vi "HW 2-1.vi"() -> ()   [LabVIEW 2017]
panel:
  in  "%":bool
  in  "+/-":bool
  in  ".":bool
  in  "blackspace":bool
  in  "ce":bool
  in  "c":bool
  in  "/":bool
  out "String":string
  in  "=":bool
  in  "c":bool
  in  "*":bool
  in  "-":bool
  in  "+":bool
  in  "9":bool
  in  "8":bool
  in  "7":bool
  in  "6":bool
  in  "5":bool
  in  "4":bool
  in  "3":bool
  in  "2":bool
  in  "1":bool
  in  "0":bool
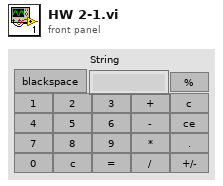
[diagram p1: front panel]
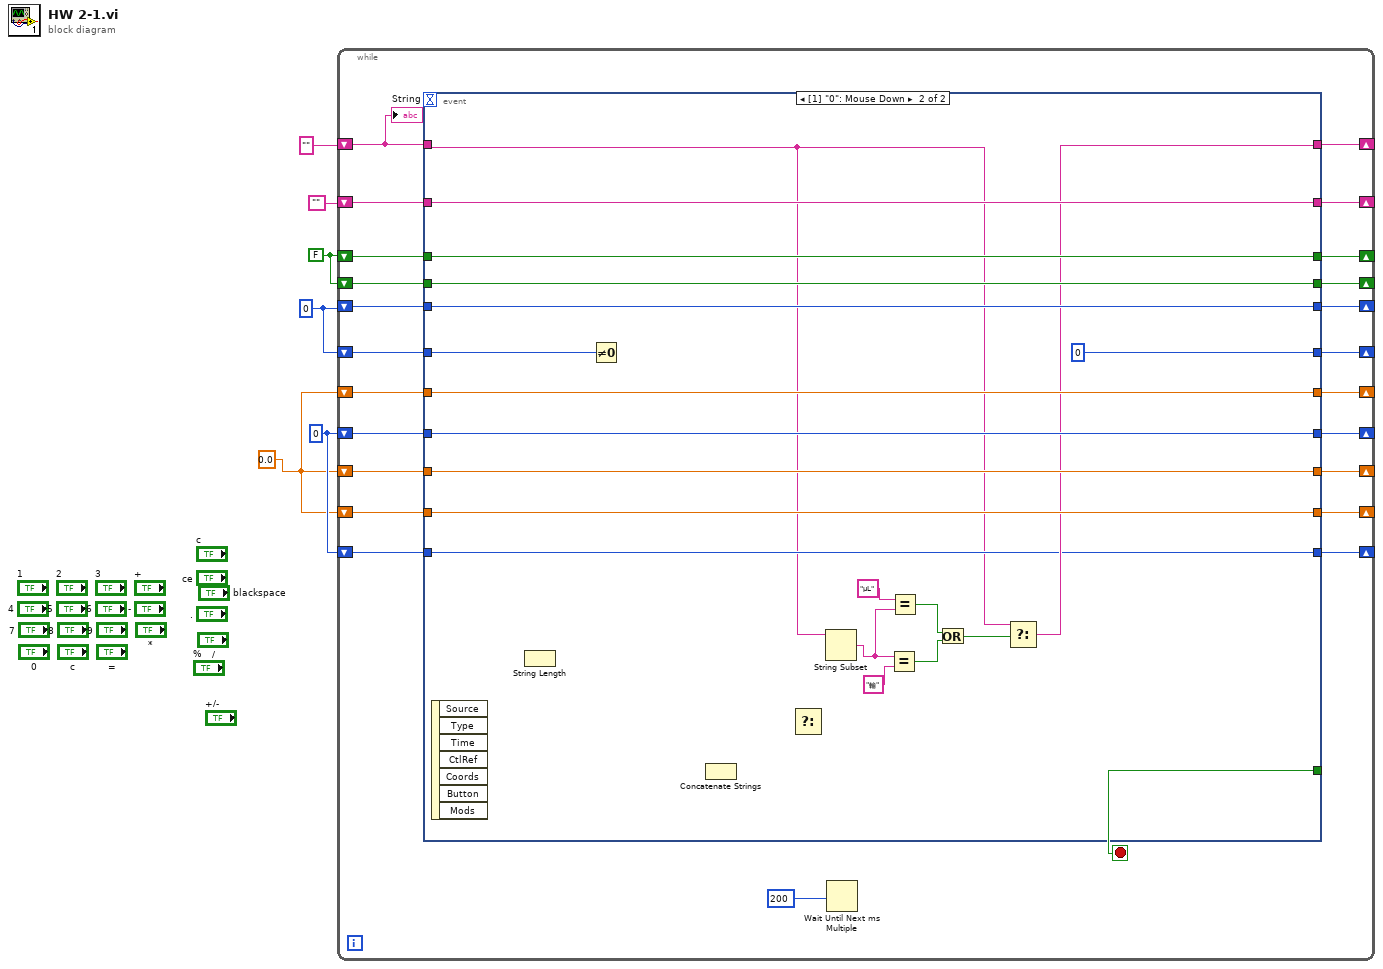
[diagram p0: block diagram]
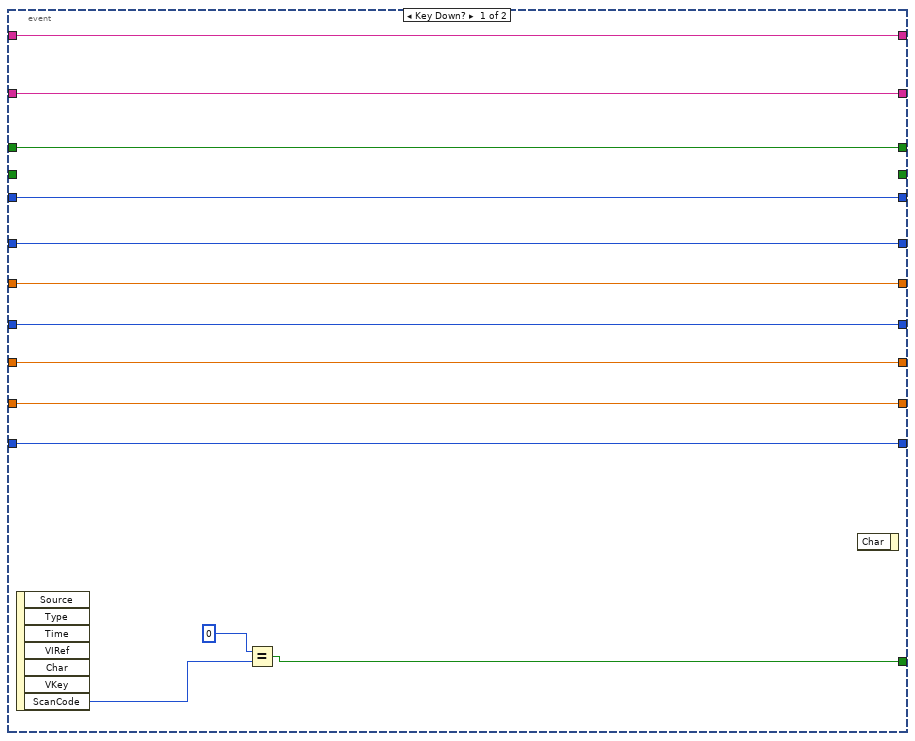
[diagram p2: hidden frame]
diagram:
  w2 = 0.0
  w3 = 0
  w4 = 0
  w1 = FALSE
  n1 = while {
    shift-right: [w30] -> _
    shift-left: "" -> [w11]
    shift-right: [w28] -> _
    shift-left: "" -> [w29]
    shift-right: [w26] -> _
    shift-left: w1 -> [w27]
    shift-right: [w24] -> _
    shift-left: w4 -> [w25]
    shift-right: [w22] -> _
    shift-left: w4 -> [w23]
    shift-right: [w20] -> _
    shift-left: w2 -> [w21]
    shift-right: [w15] -> _
    shift-left: w3 -> [w19]
    shift-right: [w14] -> _
    shift-left: w2 -> [w18]
    shift-right: [w13] -> _
    shift-left: w2 -> [w17]
    shift-right: [w12] -> _
    shift-left: w3 -> [w16]
    shift-right: [w8] -> _
    shift-left: w1 -> [w9]
    stop <- w10 stop-if-true
    n2 = event shown="[1] \"0\": Mouse Down" {
      selector: _ -> [_ _]
      dyn-events: _ -> [_ _]
      timeout: _ -> [_ _]
      tunnel: w11 -> [w43 w44]
      tunnel: [w43 w52] -> w30
      tunnel: w29 -> [w42 w62]
      tunnel: [w42 w62] -> w28
      tunnel: w27 -> [w41 w61]
      tunnel: [w41 w61] -> w26
      tunnel: w25 -> [w40 w60]
      tunnel: [w40 w60] -> w24
      tunnel: w23 -> [w39 w53]
      tunnel: [w39 0] -> w22
      tunnel: w21 -> [w38 w59]
      tunnel: [w38 w59] -> w20
      tunnel: w19 -> [w37 w58]
      tunnel: w18 -> [w36 w57]
      tunnel: w17 -> [w35 w56]
      tunnel: w16 -> [w34 w51]
      tunnel: [w37 w58] -> w15
      tunnel: [w36 w57] -> w14
      tunnel: [w35 w56] -> w13
      tunnel: [w34 w51] -> w12
      tunnel: [w31 _] -> w10
      tunnel: w9 -> [_ w55]
      tunnel: [_ w55] -> w8
      event Key Down? {
        n3 = event-data() -> ("ScanCode"=w32:i16)  [unwired: 1 in, 6 out]
        n4 = Equal?(x=0, y=w32) -> (x = y?=w31:bool)
        n5 = event-data() -> ()  [unwired: 2 in, 1 out]
      }
      event "0": Mouse Down {
        n6 = event-data() -> ()  [unwired: 1 in, 7 out]
        n7 = String Length() -> ()  [unwired: 1 in, 1 out]
        n8 = Not Equal To 0?(x=w53) -> ()  [unwired: 1 out]
        n9 = Concatenate Strings() -> ()  [unwired: 2 in, 1 out]
        n10 = Select() -> ()  [unwired: 3 in, 1 out]
        n11 = String Subset(string=w44) -> (substring=w45:string)  [unwired: 2 in]
        n12 = Equal?(x=w45, y="輸") -> (x = y?=w48:bool)
        n13 = Equal?(x="µL", y=w45) -> (x = y?=w49:bool)
        n14 = Or(x=w49, y=w48) -> (x .or. y?=w50:bool)
        n15 = Select(t=w44, s=w50) -> (s? t:f=w52:string)  [unwired: 1 in]
      }
    }
    n16 = Wait Until Next ms Multiple(millisecond multiple=u32 200 ("millisecond timer value")) -> ()  [unwired: 1 out]
    "String" <- w11
  }
